vi "PB Init.vi"(3 "Container State":T4, 4 "Previous State":variant, 5 "Previous Version":T3) -> (2 "Current State":T1={"Window Handle"=refnum, "Maximum"=100, "State Change Action"=enum."Method - Initialize", "Running"=FALSE, "Visable Items"={"Label"=TRUE, "Caption"=FALSE}, "Value"=100, "Show Progress Bar"=FALSE})   [LabVIEW 2011, in "Taskbar Progress Bar.xctl"]
uses:
  Taskbar Progress Bar.xctl
  PB State.ctl
  TypeDefs/Dispaly State Change Methods.ctl
  <vilib>/_xctls/Container State.ctl
  <vilib>/_xctls/Version.ctl
  <vilib>/_xctls/XControlSupport.lvlib
panel:
  in  "Default Indicator State":T1={"Window Handle"=refnum, "Maximum"=100, "State Change Action"=enum."Created", "Running"=FALSE, "Visable Items"={"Label"=TRUE, "Caption"=FALSE}, "Value"=100, "Show Progress Bar"=FALSE}
  in  "Default Control State":T1={"Window Handle"=refnum, "Maximum"=100, "State Change Action"=enum."Created", "Running"=FALSE, "Visable Items"={"Label"=TRUE, "Caption"=FALSE}, "Value"=100, "Show Progress Bar"=FALSE}
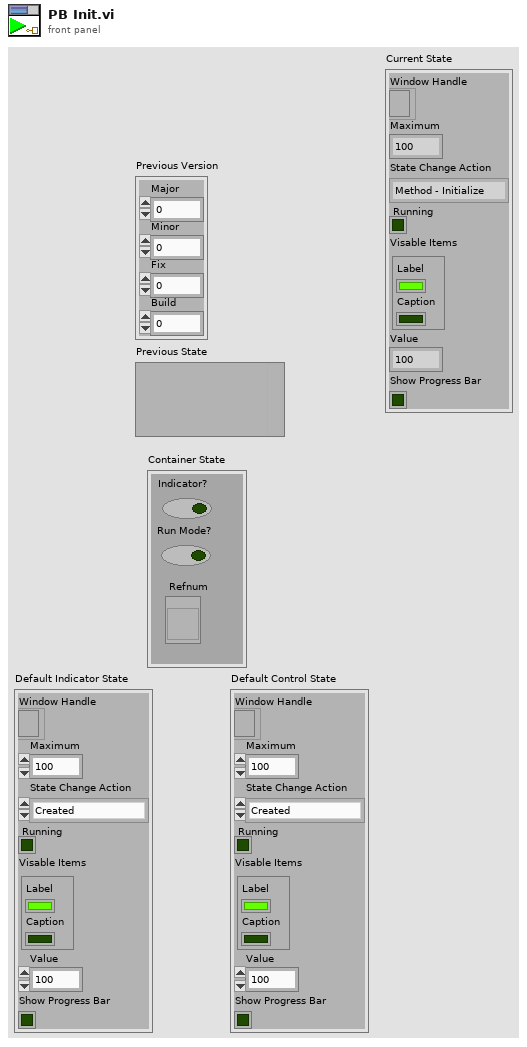
[diagram p1: front panel]
types:
  T1 = typedef "Taskbar Progress Bar.xctl/PB State.ctl" = cluster{"Window Handle":refnum<k24>, "Maximum":u64, "State Change Action":T2, "Running":bool, "Visable Items":cluster{"Label":bool, "Caption":bool}, "Value":u64, "Show Progress Bar":bool}
  T2 = typedef "Taskbar Progress Bar.xctl/Dispaly State Change Methods.ctl" = enum16{"No Action", "Created", "Method - Initialize", "Method - Increment", "Method - Pause", "Method - Error", "Method - Finish", "Property - Show Progress Bar"}
  T3 = typedef "XControlSupport.lvlib/Version.ctl" = cluster{"Major":u16, "Minor":u16, "Fix":u16, "Build":u16}
  T4 = typedef "XControlSupport.lvlib/Container State.ctl" = cluster{"Indicator?":bool, "Run Mode?":bool, " Refnum":refnum<vi>}
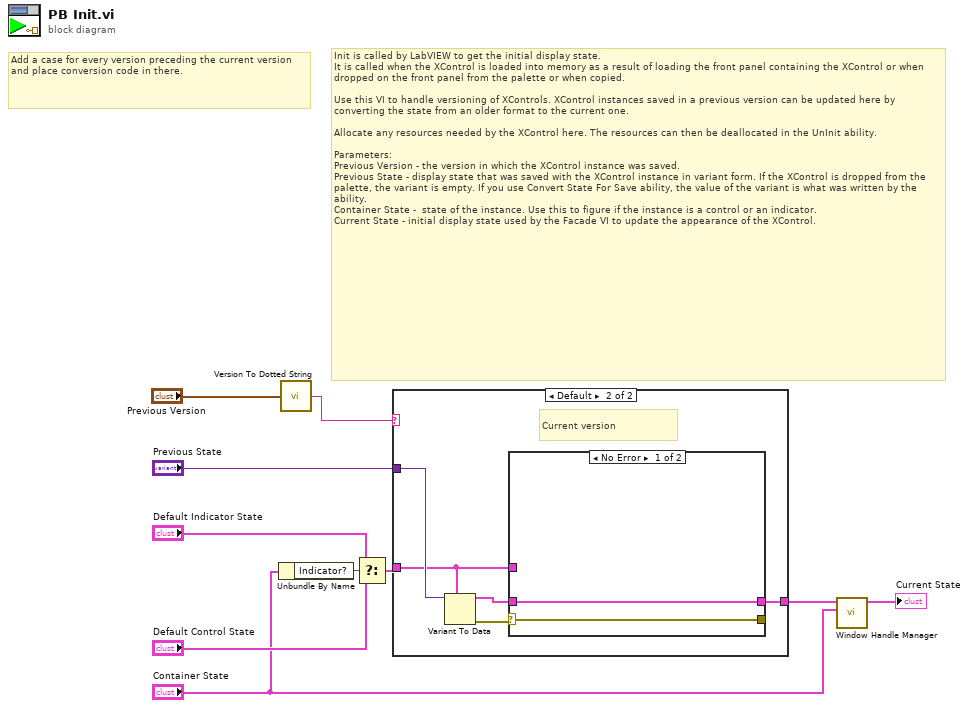
[diagram p0: block diagram]
diagram:
  # "Add a case for every version preceding the current version and place conversion code in there."
  # "Init is called by LabVIEW to get the initial display state.\nIt is called when the XControl is loaded into memory as a result of loading the front panel containing the XControl or when dropped on the front panel from the palette or when copied.\n\nUse this VI to handle versioning of XControls. XControl instances saved in a previous version can be updated here by converting the state from an older format to the current one.\n\nAllocate any resources needed by the XControl here. The resources can then be deallocated in the UnInit ability.\n\nParameters:\nPrevious Version - the version in which the XControl instance was saved.\nPrevious State - display state that was saved with the XControl instance in variant form. If the XControl is dropped from the palette, the variant is empty. If you use Convert State For Save ability, the value of the variant is what was written by the ability. \nContainer State -  state of the instance. Use this to figure if the instance is a control or an indicator.\nCurrent State - initial display state used by the Facade VI to update the appearance of the XControl."
  n1 = Unbundle By Name("Container State") -> ("Indicator?"=w7:bool)
  n2 = call <vilib>:"Version To Dotted String.vi"("Version"="Previous Version") -> ("String Version"=w4:string)
  n3 = Select(t="Default Indicator State", s=w7, f="Default Control State") -> (s? t:f=w6:T1)
  n4 = case shown="Default" w4 {
    tunnel: "Previous State" -> [_ w16]
    tunnel: [w11 w12] -> w3
    tunnel: w6 -> [w11 w13]
    frame "0.0.0.0" {
      # "Just created, use default state"
    }
    frame Default {
      # "Current version"
      n5 = Variant To Data(type=w13, Variant=w16) -> (data=w14:T1, error out=w15:errorcluster)  [unwired: 1 in]
      n6 = case shown="No Error" w15 {
        selector: w15 -> [w18 w19]
        tunnel: w14 -> [w17 _]
        tunnel: [w17 w20] -> w12
        tunnel: w13 -> [_ w20]
        tunnel: [w18 w19] -> _
        frame No Error {
        }
        frame Error {
          # "Error converting previously \nsaved state. Use default instead."
        }
      }
    }
  }
  n7 = call "Window Handle Manager.vi"("Container State"="Container State", "Display State in"=w3) -> ("Display State out"=→"Current State":T1)  [unwired: 9 in]
